vi "GUI step til data step.vi"(7 "GUI step clluster":T1) -> (8 "data step cluster":T5)   [LabVIEW 2011]
uses:
  Sequence steps config..ctl
  Single criteria cluster.ctl
  Criteria types.ctl
  Boolean operation.ctl
  Sequence step GUI.ctl
  X-cont Action select/Action select.xctl
  X-cont criteria/Criteria control.xctl
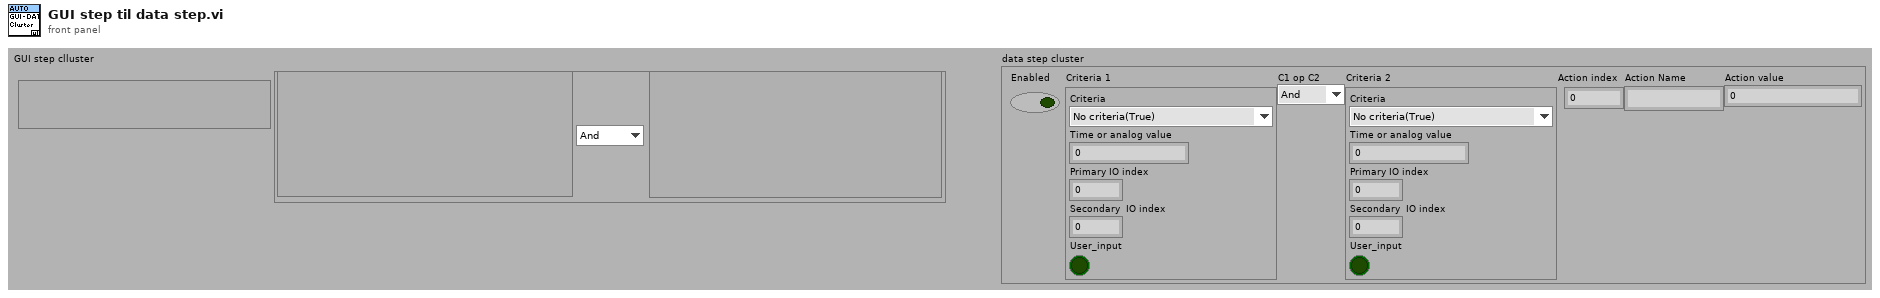
[diagram p1: front panel]
types:
  T1 = typedef "Sequence step GUI.ctl" = cluster{"Action select":cluster{"Action index":i32, "Data":dbl}, "Criteria 1":cluster{"Criteria":T2}, "C1 op C2":T4, "Criteria 2":cluster{"Criteria":T2}}
  T2 = typedef "Single criteria cluster.ctl" = cluster{"Criteria":T3, "Time or analog value":dbl, "Primary IO index":i32, "Secondary  IO index":i32, "User_input":bool}
  T3 = typedef "Criteria types.ctl" = enum16{"No criteria(True)", "Time(s)", "Analog IO over", "Analog IO over or equal", "Analog IO under", "Analog IO under or equal", "Analog IO 1 minus Analog IO 2 over", "Digital IO True", "Digital IO False", "Operator approval"}
  T4 = typedef "Boolean operation.ctl" = enum16{"And", "Or", "Xor", "Nand", "Nor", "Nxor", "Implies"}
  T5 = typedef "Sequence steps config..ctl" = cluster{"Enabled":bool, "Criteria 1":T2, "C1 op C2":T4, "Criteria 2":T2, "Action index":i32, "Action Name":string, "Action value":dbl}
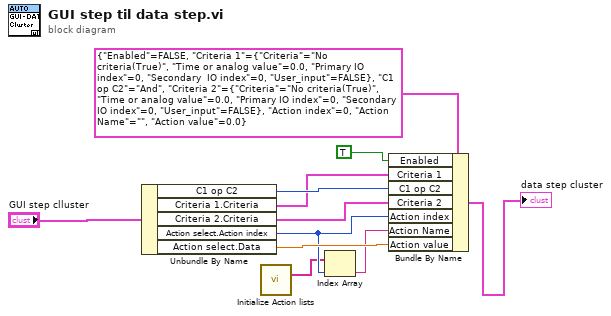
[diagram p0: block diagram]
diagram:
  n1 = Unbundle By Name("GUI step clluster") -> ("C1 op C2"=w6:T4, "Criteria 1.Criteria"=w4:T2, "Criteria 2.Criteria"=w5:T2, "Action select.Action index"=w8:i32, "Action select.Data"=w10:dbl)
  n2 = call "Initialize Action lists.vi"() -> ("Action names"=w7:string[])  [unwired: 13 in, 2 out]
  n3 = Index Array(array=w7, index=w8) -> (element=w9:string)
  n4 = Bundle By Name(cluster=T5 {"Enabled"=FALSE, "Criteria 1"={"Criteria"=enum."No criteria(True)", "Time or analog value"=0.0, "Primary IO index"=0, "Secondary  IO index"=0, "User_input"=FALSE}, "C1 op C2"=enum."And", "Criteria 2"={"Criteria"=enum."No criteria(True)", "Time or analog value"=0.0, "Primary IO index"=0, "Secondary  IO index"=0, "User_input"=FALSE}, "Action index"=0, "Action Name"="", "Action value"=0.0} ("Sequence step config"), "Enabled"=TRUE, "Criteria 1"=w4, "C1 op C2"=w6, "Criteria 2"=w5, "Action index"=w8, "Action Name"=w9, "Action value"=w10) -> (→"data step cluster":T5)
